vi "Log Data.vi"(8 "error in (no error)":errorcluster, 10 "Data Queue":T1, 11 "Logging Configuration":T2) -> (0 "error out":errorcluster)   [LabVIEW 2021, in "IMU Logging.lvlib"]
doc: "This VI uses the TDMS Write function to write data to a TDMS file."
uses:
  IMU Logging.lvlib
  Logging Configuration.ctl
  Acquisition/IMU Data Queue.ctl
  IMU TimeDataStruct.ctl
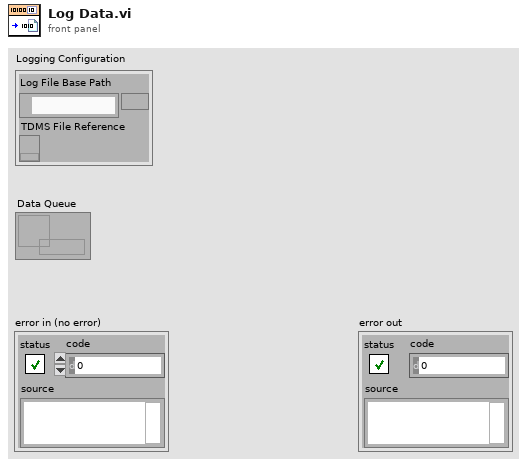
[diagram p1: front panel]
types:
  T1 = typedef "IMU Data Queue.ctl" = refnum<queue>
  T2 = typedef "IMU Logging.lvlib/Logging Configuration.ctl" = cluster{"Log File Base Path":path, "TDMS File Reference":refnum<k34>}
  T3 = typedef "IMU TimeDataStruct.ctl" = cluster{string, dbl[]}
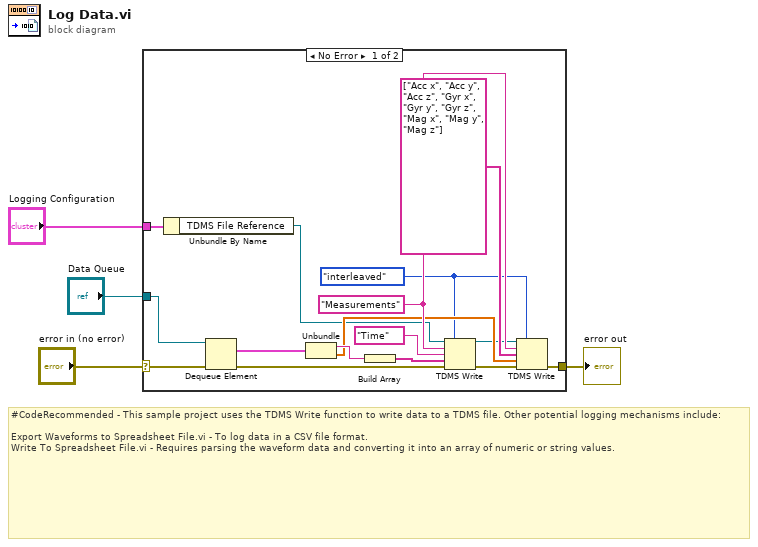
[diagram p0: block diagram]
diagram:
  # "#CodeRecommended - This sample project uses the TDMS Write function to write data to a TDMS file. Other potential logging mechanisms include:\n\nExport Waveforms to Spreadsheet File.vi - To log data in a CSV file format.\nWrite To Spreadsheet File.vi - Requires parsing the waveform data and converting it into an array of numeric or string values."
  n1 = case shown="No Error" "error in (no error)" {
    selector: "error in (no error)" -> [w19 w21]
    tunnel: "Logging Configuration" -> [w20 _]
    tunnel: "Data Queue" -> [w18 _]
    tunnel: [w8 w21] -> w2
    frame No Error {
      w17 = "Measurements" ("group name in (Untitled)")
      w5 = enum16{"decimated", "interleaved"}."interleaved" ("data layout (0:decimated)")
      n2 = Unbundle By Name(w20) -> ("TDMS File Reference"=w7:refnum<k34>)
      n3 = Dequeue Element(queue=w18, error in (no error)=w19) -> (element=w15:T3, error out=w10:errorcluster)  [unwired: 1 in, 2 out]
      n4 = Unbundle(w15) -> (w16:string, w14:dbl[])
      n5 = Build Array(w16) -> (w13:string[])
      n6 = TDMS Write(0:w7, 1:w5, 5:w17, 7:"Time" ("channel name(s) in (Untitled)"), 9:w13, 11:w10) -> (4:w6:refnum<k34>, 15:w9:errorcluster)  [unwired: 2 out]
      n7 = TDMS Write(0:w6, 1:w5, 5:w17, 7:string[] ["Acc x", "Acc y", "Acc z", "Gyr x", "Gyr y", "Gyr z", "Mag x", "Mag y", "Mag z"] ("channel name(s) in (Untitled)"), 9:w14, 11:w9) -> (15:w8:errorcluster)  [unwired: 3 out]
    }
    frame Error {
    }
  }
  "error out" <- w2
